vi "Speed controls.vi"() -> ()   [LabVIEW 2018]
uses:
  <vilib>/Platform/TimedLoop/XDataNode/timing_clust.ctl
  <vilib>/Platform/TimedLoop/XDataNode/nitl_modes.ctl
  <vilib>/Platform/TimedLoop/XDataNode/wakeup.ctl
  <vilib>/platform/TimedLoop/XDataNode/XDataNode.xnode
  <vilib>/Platform/TimedLoop/XDataNode/XDNodeRunTimeDep.lvlib
panel:
  in  "stop":bool
  in  "power":dbl
  out "Encorder":dbl[](array[numeric])
  in  "Reset":bool
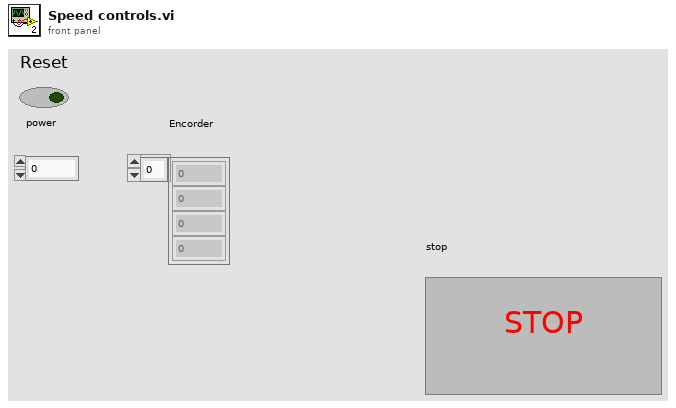
[diagram p1: front panel]
types:
  T1 = typedef "XDNodeRunTimeDep.lvlib/timing_clust.ctl" = cluster{"Expected End [f-1]":u64, "Actual End [f-1]":u64, "Finished Late? [f-1]":bool, "Expected End [i-1]":u64, "Actual End [i-1]":u64, "Finished Late? [i-1]":bool, "Expected Start [i]":u64, "Actual Start [i]":u64, "Expected Start [f]":u64, "Actual Start [f]":u64, "Source Name":string, "Structure Name":string, "Period":i64, "Deadline":i64, "Offset":i64, "Start":i64, "Priority":i32, "Timeout":i32, "Mode":T2, "Wakeup Reason":T3, "Error":errorcluster, "Source Type":string, "Secondary Source Type":string, "Global End Time":u64, "Global Start Time":u64, "Frame Duration":u64, "Iteration Duration":u64, "Assigned CPU":i32, "I/O Scan Engine Mode":u32}
  T2 = typedef "XDNodeRunTimeDep.lvlib/nitl_modes.ctl" = enum32{"No Change", "Process missed periods, maintain original phase", "Discard missed periods, maintain original phase", "Process missed periods, ignore original phase", "Discard missed periods, ignore original phase"}
  T3 = typedef "XDNodeRunTimeDep.lvlib/wakeup.ctl" = enum32{"Normal", "Aborted", "Asynchronous wakeup", "Timing source error", "Timed loop error", "Timeout"}
  T4 = cluster{"proportional gain (Kc)":dbl, "integral time (Ti, min)":dbl, "derivative time (Td, min)":dbl}
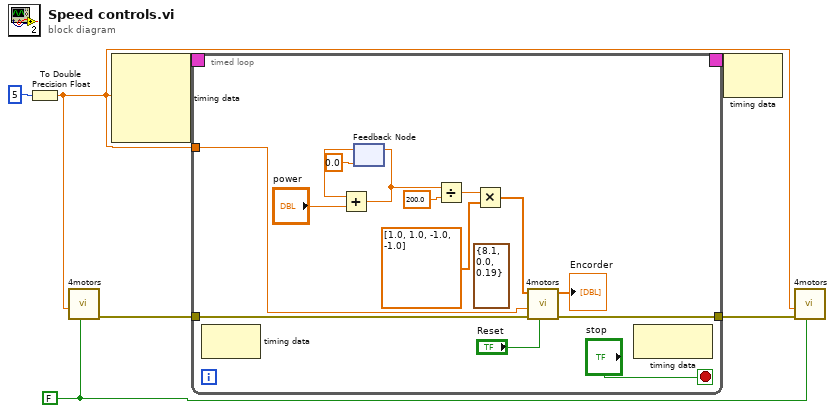
[diagram p0: block diagram]
diagram:
  w5 = FALSE ("Reset")
  n1 = To Double Precision Float(number=i64 5 ("Period")) -> (double precision float=w1:dbl)
  n2 = call "4motors.vi"("Reset"=w5, "dt(s)"=w1) -> ("error out"=w4:errorcluster)  [unwired: 8 in, 1 out]
  n3 = node-c288(w1) -> (w7:T1)  [unwired: 3 in]
  n4 = timed-loop {
    timing: w7 -> [_]
    timing-out: [_] -> w6
    tunnel: w1 -> [w10]
    tunnel: w4 -> [w20]
    tunnel: [w19] -> w3
    stop <- "stop" stop-if-true
    (unwired) T4 {"proportional gain (Kc)"=8.1, "integral time (Ti, min)"=0.0, "derivative time (Td, min)"=0.19} ("PID gains")
    n5 = node-c288() -> ()  [unwired: 1 in, 1 out]
    n6 = feedback #1(0.0) -> (w17:dbl)
    n7 = Add(x=w17, y="power") -> (x+y=w9:dbl)
    n8 = feedback-in #1(w9) -> ()
    n9 = Divide(x=w9, y=200.0) -> (x/y=w8:dbl)
    n10 = Multiply(x=w8, y=dbl[] [1.0, 1.0, -1.0, -1.0]) -> (x*y=w14:dbl[])
    n11 = call "4motors.vi"("Reset"="Reset", "error in (no error)"=w20, "dt(s)"=w10, "Power"=w14) -> ("error out"=w19:errorcluster, "Encorder"=→"Encorder":dbl[])  [unwired: 6 in]
    n12 = node-c288() -> ()  [unwired: 1 in, 1 out]
  }
  n13 = node-c288(w6) -> ()  [unwired: 1 out]
  n14 = call "4motors.vi"("Reset"=w5, "error in (no error)"=w3, "dt(s)"=w1) -> ()  [unwired: 7 in, 2 out]
